vi "Find VI on Disk by Node.vi"() -> ()   [LabVIEW 2020]
uses:
  _Node Names.ctl
panel:
  in  "Tab Control":enum32{"Settings", "Results", "Text Results"}(tab)
  in  "Search":bool
  out "Current directory/llb":path
  in  "pattern":string="*.vi"
  in  "Directory to search":path=path "C:/Program Files/National Instruments/LabVIEW 8.2/vi.lib/addons/Simulation Interface"
  in  "Class Name":T1="Invoke"
  in  "Item Name (method or property)":string="Create Constant"
  out "Found":path[](array[path])
  out "String":string
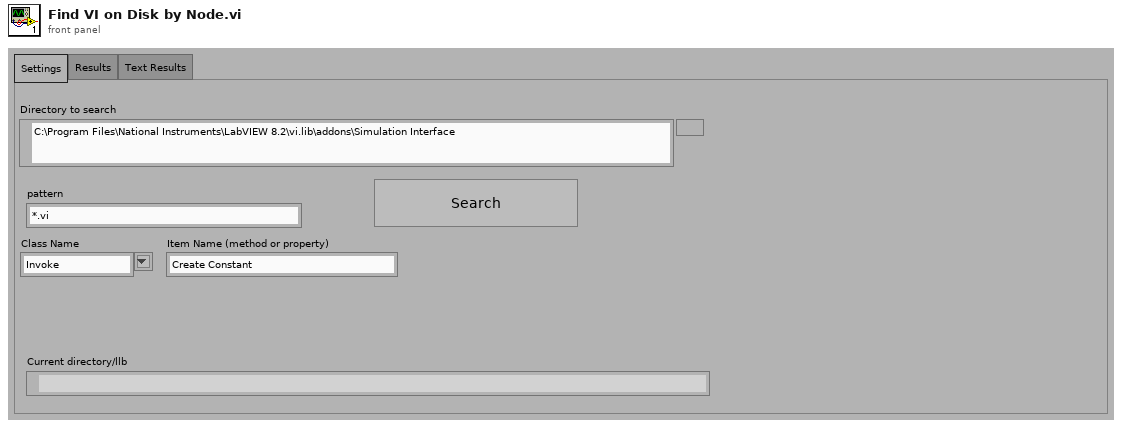
[diagram p1: front panel]
types:
  T1 = typedef "_Node Names.ctl" = string
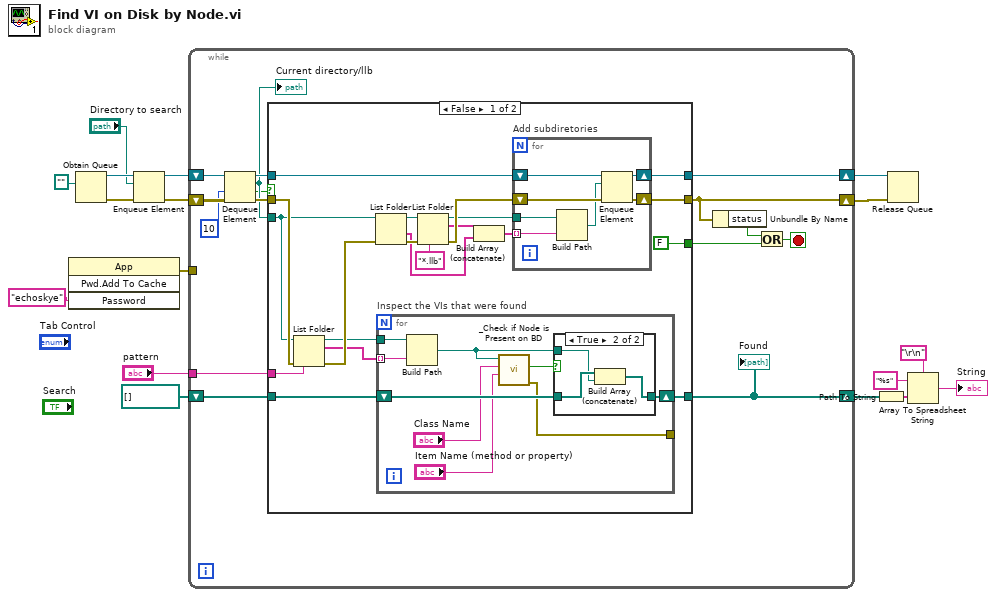
[diagram p0: block diagram]
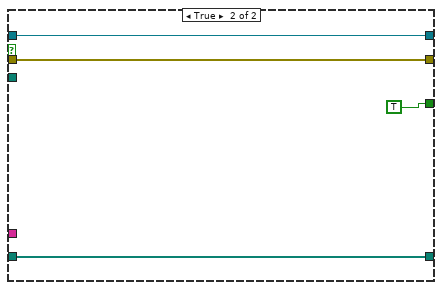
[diagram p3: hidden frame]
diagram:
  n1 = invoke class="App" method="Pwd.Add To Cache"("Password"="echoskye") -> (error out=w6:errorcluster)  [unwired: 3 in, 3 out]
  n2 = Obtain Queue(element data type=path "") -> (queue out=w16:refnum<queue>, error out=w15:errorcluster)  [unwired: 4 in, 1 out]
  n3 = Enqueue Element(queue=w16, element="Directory to search", error in (no error)=w15) -> (queue out=w13:refnum<queue>, error out=w12:errorcluster)  [unwired: 1 in, 1 out]
  n4 = while {
    shift-right: [w29] -> w5
    shift-left: path[] [] -> [w28]
    shift-right: [w26] -> w11
    shift-left: w13 -> [w31]
    shift-right: [w21] -> w10
    shift-left: w12 -> [w32]
    tunnel: "pattern" -> [w23]
    tunnel: w6 -> [_]
    stop <- w19 stop-if-true
    n5 = Dequeue Element(queue=w31, timeout in ms (-1)=10, error in (no error)=w32) -> (queue out=w27:refnum<queue>, element=w24:path, timed out?=w22:bool, error out=w25:errorcluster)
    "Current directory/llb" <- w24
    n6 = case shown="False" w22 {
      tunnel: [w38 w75] -> w29
      tunnel: w28 -> [w39 w75]
      tunnel: w27 -> [w51 w76]
      tunnel: [w50 w76] -> w26
      tunnel: w25 -> [w49 w74]
      tunnel: [w48 w74] -> w21
      tunnel: w24 -> [w36 _]
      tunnel: w23 -> [w41 _]
      tunnel: [FALSE TRUE] -> w18
      frame False {
        n7 = List Folder(path=w36, pattern=w41, error in=w49) -> (path out=w37:path, filenames=w40:string[], error out=w52:errorcluster)  [unwired: 1 in, 1 out]
        n8 = List Folder(path=w36, error in=w52) -> (path out=w35:path, folder names=w44:string[], error out=w45:errorcluster)  [unwired: 2 in, 1 out]
        n9 = for "Inspect the VIs that were found" {
          tunnel: w37 -> [w61]
          tunnel: w40 -> [w60] mode=indexing
          shift-right: [w56] -> w38
          shift-left: w39 -> [w57]
          tunnel: [w53] -> _
          n10 = Build Path(base path=w61, name or relative path=w60) -> (appended path=w59:path)
          n11 = call "_Check if Node is Present on BD.vi"("Name of Selection"="Item Name (method or property)", "Class Name"="Class Name", "path"=w59) -> ("error out"=w53:errorcluster, "Found?"=w58:bool)  [unwired: 7 in]
          n12 = case shown="True" w58 {
            tunnel: w57 -> [w62 w65]
            tunnel: w59 -> [_ w64]
            tunnel: [w62 w63] -> w56
            frame False {
            }
            frame True {
              n13 = Build Array (concatenate)(w65, w64) -> (w63:path[])
            }
          }
        }
        n14 = List Folder(path=w35, pattern="*.llb", error in=w45) -> (path out=w34:path, filenames=w43:string[], error out=w46:errorcluster)  [unwired: 1 in, 1 out]
        n15 = Build Array (concatenate)(w43, w44) -> (w42:string[])
        n16 = for "Add subdiretories" {
          tunnel: w42 -> [w72] mode=indexing
          tunnel: w34 -> [w71]
          shift-right: [w67] -> w48
          shift-left: w46 -> [w70]
          shift-right: [w66] -> w50
          shift-left: w51 -> [w69]
          n17 = Build Path(base path=w71, name or relative path=w72) -> (appended path=w68:path)
          n18 = Enqueue Element(queue=w69, element=w68, error in (no error)=w70) -> (queue out=w66:refnum<queue>, error out=w67:errorcluster)  [unwired: 1 in, 1 out]
        }
      }
      frame True {
      }
    }
    "Found" <- w29
    n19 = Unbundle By Name(w21) -> ("status"=w20:bool)
    n20 = Or(x=w20, y=w18) -> (x .or. y?=w19:bool)
  }
  n21 = Path To String(path=w5) -> (string=w4:string[])
  n22 = Release Queue(queue=w11, error in (no error)=w10) -> ()  [unwired: 1 in, 3 out]
  n23 = Array To Spreadsheet String(delimiter (Tab)="\r\n", array=w4, 3:"%s" ("format string")) -> (spreadsheet string=→"String":string)
